vi "EjerciciodeWhile_Curso.vi"() -> ()   [LabVIEW 2022 SP3]
panel:
  out "Numeric 2":i32
  in  "Numeric":i32
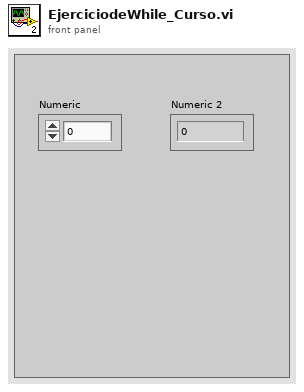
[diagram p1: front panel]
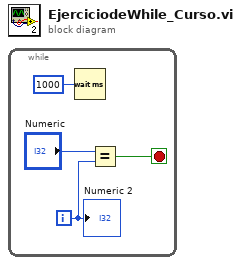
[diagram p0: block diagram]
diagram:
  n1 = while {
    i -> [w3]
    stop <- w2 stop-if-true
    n2 = Wait (ms)(milliseconds to wait=u32 1000) -> ()  [unwired: 1 out]
    n3 = Equal?(x="Numeric", y=w3) -> (x = y?=w2:bool)
    "Numeric 2" <- w3
  }
